vi "Config.Add SW Item.vi"(6 "Note":string, 8 "Version":string, 9 "PN":string, 10 "Name":string, 11 "SW List In":string[][](array[string])) -> (1 "Modified":bool, 3 "SW List Out":string[][](array[string]))   [LabVIEW 2024, in "EQMF.lvlib" / "Config Utils.lvlib"]
doc: "This VI inputs a 2D array of string that is the SW item list and appends an item.\nEach row of the 2D array is a SW item record.\nThe columns are: Name, PN, Version, Notes\n\nIf a record already exists with the same Name, then that record will eb replaced with the new SW item.\n\nINPUTS:\n<B>Name</B> - Name of the SW item.\n<B>PN</B> - Part Number of the SW item.\n<B>Version</B> - Version of the SW item.\n<B>Note</B> - Any notes related to the SW item.\n\nOUTPUTS:\n<B>Modified</B> - TRUE indicates the name was already in the SW item list and that record has been updated.\n\nERRORS: \nN/A"
uses:
  Config Utils.lvlib
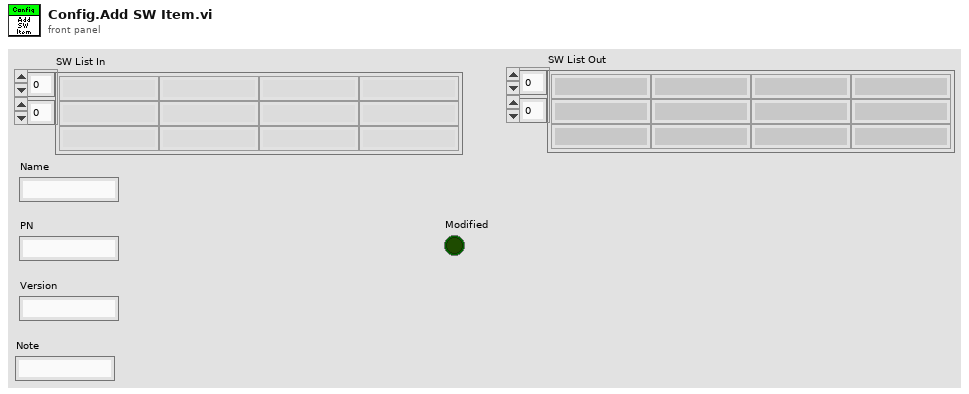
[diagram p1: front panel]
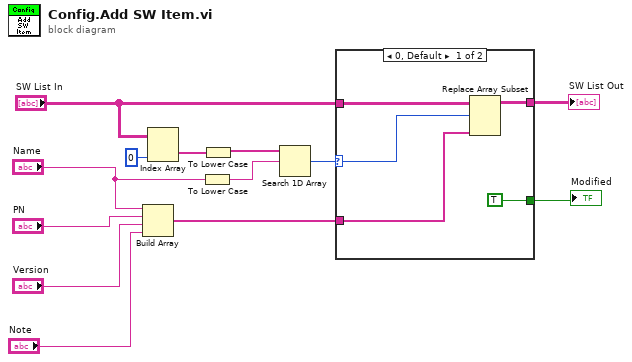
[diagram p0: block diagram]
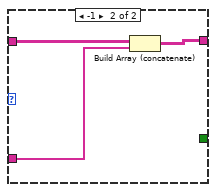
[diagram p2: hidden frame]
diagram:
  n1 = Build Array("Name", "PN", "Version", "Note") -> (w2:string[])
  n2 = Index Array(array="SW List In", index (col)=0 ("index")) -> (element=w9:string[])  [unwired: 1 in]
  n3 = To Lower Case(string="Name") -> (all lower case string=w6:string)
  n4 = To Lower Case(string=w9) -> (all lower case string=w7:string[])
  n5 = Search 1D Array(1D array=w7, element=w6) -> (index of element=w5:i32)  [unwired: 1 in]
  n6 = case shown="0, Default" w5 {
    selector: w5 -> [w16 _]
    tunnel: "SW List In" -> [w18 w21]
    tunnel: [w17 w20] -> w3
    tunnel: w2 -> [w15 w19]
    tunnel: [TRUE _] -> w1
    frame 0, Default {
      n7 = Replace Array Subset(array=w18, new element=w15, index (row)=w16) -> (w17:string[][])  [unwired: 1 in]
    }
    frame -1 {
      n8 = Build Array (concatenate)(w21, w19) -> (w20:string[][])
    }
  }
  "SW List Out" <- w3
  "Modified" <- w1
